vi "Build Messages.vi"(8 "error in (no error)":errorcluster, 11 "Bus Controller XML Node":refnum<k20>) -> (0 "error out":errorcluster, 3 "Messages":refnum<class "Message.lvclass">[](array[class]))   [LabVIEW 2016]
doc: "Builds all the Messages defined in the BCMessages XML node. Each Message should have a unique name property."
uses:
  <vilib>/xml/NI_XML.lvlib
  Frames & Messages/RT-RT Message/RT-RT Message.lvclass
  Frames & Messages/Message/Message.lvclass
  D:/SVN/Products/BCI-1553/Software/Development/2016/RealTime/Driver (Windows)/Frames & Messages/Message/Message.lvclass
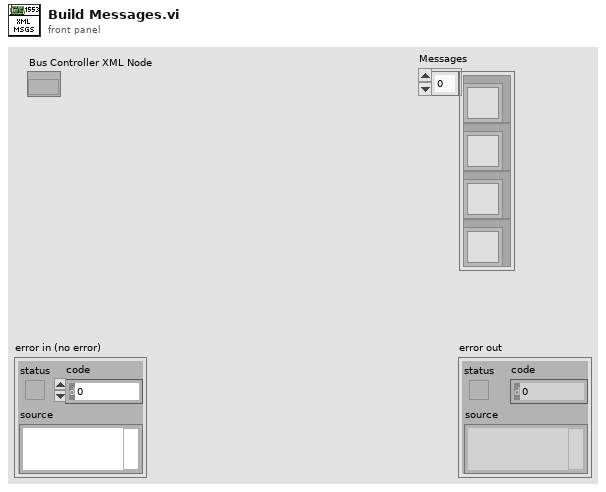
[diagram p1: front panel]
types:
  T1 = typedef "BCI-1553 API.lvlib/Message Config.ctl" = cluster{"Time to Next Msg (4 us)":u16, "Command Config":T2, "Message Control":T3}
  T2 = typedef "BCI-1553 API.lvlib/Command Config.ctl" = cluster{"Command Type":enum16{"Transmit", "Receive"}, "Terminal Address (0-30)":u16, "SubAddress (1-30)":u16, "WC/MC (1-32)":u16, "Command Data":u16[]}
  T3 = typedef "BCI-1553 API.lvlib/Message Control.ctl" = cluster{"MC17 Time Sync":bool, "Error Mask":bool, "Service Request Mask":bool, "Busy Mask":bool, "SubSystem Flag Mask":bool, "Terminal Flag Mask":bool, "Reserved Mask":bool, "Retry":bool, "Bus A / !Bus B":bool, "Self-Test Loopback":bool, "Broadcast Mask":bool, "EoM Interrupt":bool, "Mode Code Format":bool, "Broadcast Format":bool, "RT-RT Format":bool}
  T4 = typedef "BCI-1553 API.lvlib/RT-RT Message Config.ctl" = cluster{"Tx Command Config":T2}
  T5 = typedef "BCI-1553 API.lvlib/1553 SubComponent.lvclass/Parameter Table Data.ctl" = cluster{"Parameter Name":string, "Base Word":u16, "Address":u16, "Value":u64, "Mask":u16[], "Scaling Info":T6}
  T6 = typedef "BCI-1553 API.lvlib/1553 SubComponent.lvclass/Scaling Information.ctl" = cluster{"Bit Offset":i32, "Bit Count":i32, "LSB Resolution":dbl, "2's Complement":bool, "Big Endian":bool, "Sign Bit":bool}
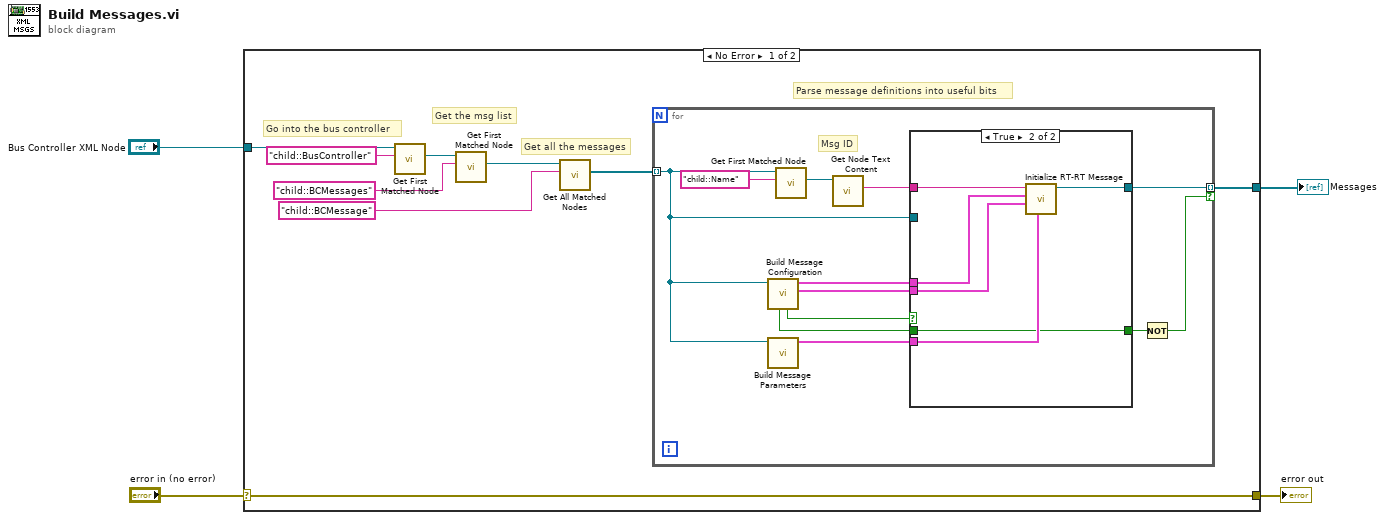
[diagram p0: block diagram]
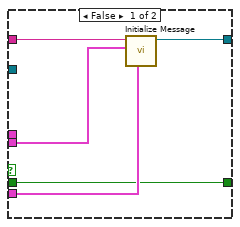
[diagram p2: hidden frame]
diagram:
  n1 = case shown="No Error" "error in (no error)" {
    selector: "error in (no error)" -> [w13 w37]
    tunnel: [w13 w37] -> w3
    tunnel: "Bus Controller XML Node" -> [w12 _]
    tunnel: [w5 _] -> w1
    frame No Error {
      # "Parse message definitions into useful bits"
      # "Get all the messages"
      # "Get the msg list"
      # "Go into the bus controller"
      n2 = call <vilib>:"Get First Matched Node.vi"("XPath expression"="child::BusController", "node in"=w12) -> ("node result"=w10:refnum<k20>)  [unwired: 7 in, 2 out]
      n3 = call <vilib>:"Get First Matched Node.vi"("XPath expression"="child::BCMessages", "node in"=w10) -> ("node result"=w8:refnum<k20>)  [unwired: 7 in, 2 out]
      n4 = call <vilib>:"Get All Matched Nodes.vi"("XPath expression"="child::BCMessage", "node in"=w8) -> ("node result array"=w6:refnum<k20>[])  [unwired: 7 in, 2 out]
      n5 = for {
        tunnel: w6 -> [w20] mode=indexing
        tunnel: [w21] -> w5 mode=indexing if=w14
        # "Msg ID"
        n6 = call "Build Message Configuration.vi"("Message XML Node"=w20) -> ("Message  Config"=w18:T1, "RT-RT Message Config"=w17:T4, "RT-RT?"=w19:bool, "Async?"=w16:bool)  [unwired: 6 in, 1 out]
        n7 = call "Build Message Parameters.vi"("Message XML Node"=w20) -> ("Parameters"=w22:T5[])  [unwired: 9 in, 1 out]
        n8 = call <vilib>:"Get First Matched Node.vi"("XPath expression"="child::Name", "node in"=w20) -> ("node result"=w24:refnum<k20>)  [unwired: 7 in, 2 out]
        n9 = call <vilib>:"Get Node Text Content.vi"("node in"=w24) -> ("node text"=w23:string)  [unwired: 8 in, 2 out]
        n10 = case shown="True" w19 {
          tunnel: w23 -> [w30 w35]
          tunnel: w22 -> [w29 w34]
          tunnel: [w28 w36] -> w21
          tunnel: w20 -> [_ _]
          tunnel: w18 -> [w27 w33]
          tunnel: w17 -> [_ w32]
          tunnel: w16 -> [w26 w31]
          tunnel: [w26 w31] -> w15
          frame False {
            n11 = call "Initialize Message.vi"("Parameters"=w29, "Message  Config"=w27, "ID"=w30) -> ("Message out"=w28:refnum<class "Message.lvclass">)  [unwired: 7 in, 1 out]
          }
          frame True {
            n12 = call "Initialize RT-RT Message.vi"("Parameters"=w34, "Message Config"=w33, "RT-RT Message Config"=w32, "ID"=w35) -> ("RT-RT Message out"=w36:refnum<class "RT-RT Message.lvclass">)  [unwired: 6 in, 1 out]
          }
        }
        n13 = Not(x=w15) -> (.not. x?=w14:bool)
      }
    }
    frame Error {
    }
  }
  "error out" <- w3
  "Messages" <- w1
